vi "Fetch Multiple Points.vi"(8 "error in (no error)":errorcluster, 9 "Timeout (10000 ms)":i32=10000 format="%#.6g", 11 "VISA resource name":refnum<visa-resource-name>) -> (0 "error out":errorcluster, 2 "Measurements":dbl[](array[numeric]), 3 "VISA resource name out":refnum<visa-resource-name>)   [LabVIEW 2013, in "Template - DMM.lvlib"]
doc: "This low-level VI returns an array of values from a previously initiated measurement. The number of measurements the DMM takes is determined by the values you specify for the <B>Trigger Count</B> control and <B>Sample Count</B> control of the Configure Multipoint VI.\n\n<B>Note:</B> Use this VI only with other low-level VIs. The high-level VIs automatically incorporate this functionality. This VI does not check the instrument status. If you want to check the instrument status, call the Error Query VI at the conclusion of the sequence."
uses:
  <instrlib>/_Template - DMM/Template - DMM.lvlib
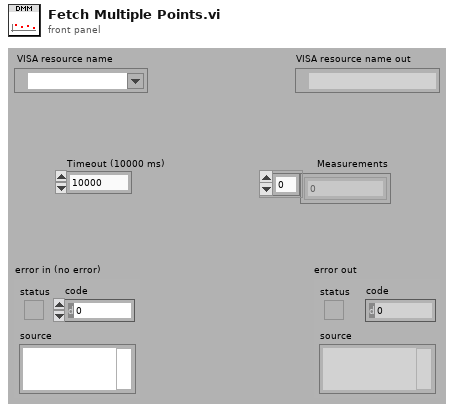
[diagram p1: front panel]
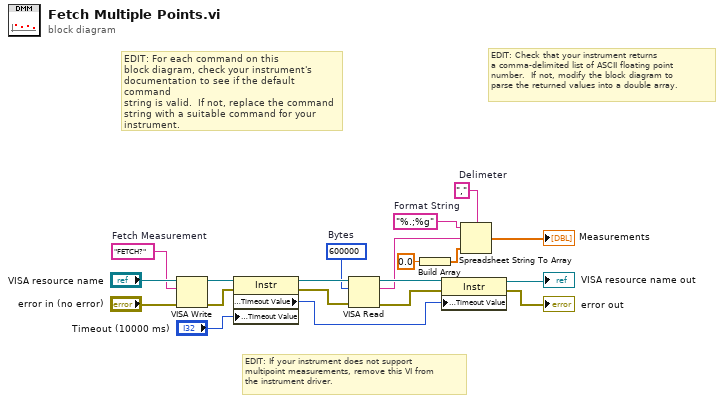
[diagram p0: block diagram]
diagram:
  w16 = ","  # Delimeter
  w17 = "%.;%g"  # Format String
  w18 = "FETCH?"  # Fetch Measurement
  w1 = u32 600000  # Bytes
  # "EDIT: If your instrument does not support\nmultipoint measurements, remove this VI from\nthe instrument driver."
  # "EDIT: Check that your instrument returns\na comma-delimited list of ASCII floating point\nnumber.  If not, modify the block diagram to\nparse the returned values into a double array."
  # "EDIT: For each command on this\nblock diagram, check your instrument's\ndocumentation to see if the default command\nstring is valid.  If not, replace the command\nstring with a suitable command for your\ninstrument."
  n1 = VISA Write(VISA resource name="VISA resource name", write buffer=w18, error in (no error)="error in (no error)") -> (VISA resource name out=w12:refnum<visa-resource-name>, error out=w11:errorcluster)  [unwired: 1 out]
  n2 = property class="Instr"(reference=w12, error in=w11, "General Settings:Timeout Value"="Timeout (10000 ms)") -> (reference out=w10:refnum<visa-resource-name>, error out=w9:errorcluster, "General Settings:Timeout Value"=w5:u32)
  n3 = VISA Read(VISA resource name=w10, byte count=w1, error in (no error)=w9) -> (VISA resource name out=w7:refnum<visa-resource-name>, read buffer=w2:string, error out=w6:errorcluster)  [unwired: 1 out]
  n4 = Build Array(0.0) -> (w14:dbl[])
  n5 = property class="Instr"(reference=w7, error in=w6, "General Settings:Timeout Value"=w5) -> (reference out=→"VISA resource name out":refnum<visa-resource-name>, error out=→"error out":errorcluster)
  n6 = Spreadsheet String To Array(delimiter (Tab)=w16, format string=w17, spreadsheet string=w2, array type (2D Dbl)=w14) -> (array=→"Measurements":dbl[])
